vi "Proj3_Wireless_DTMF_Transmitter.vi"(6 "Gray Bit Encoding":bool, 7 "Dial Tone":bool, 8 "Quantization Level":u16(ring)=4 items=["2"=2, "4"=4, "8"=8, "16"=16], 9 "Phone # String":string) -> (0 "In Transmission":bool, 1 "bitLength":i32, 2 "quants":dbl[](array[numeric]), 3 "TXbitStream":i8[](array[numeric]), 4 "TX DTMF Signal":dbl[][](array[numeric]))   [LabVIEW 2011]
panel:
  out "Transmitted DTMF Signal":dbl[][](graph)
  in  "Tab Control":enum32{"DTMF", "Quantization"}(tab)
  in  "OK Button":bool
  in  "Snapshot Run":bool=TRUE
  # "Project 3: Wireless DTMF Transmitter"
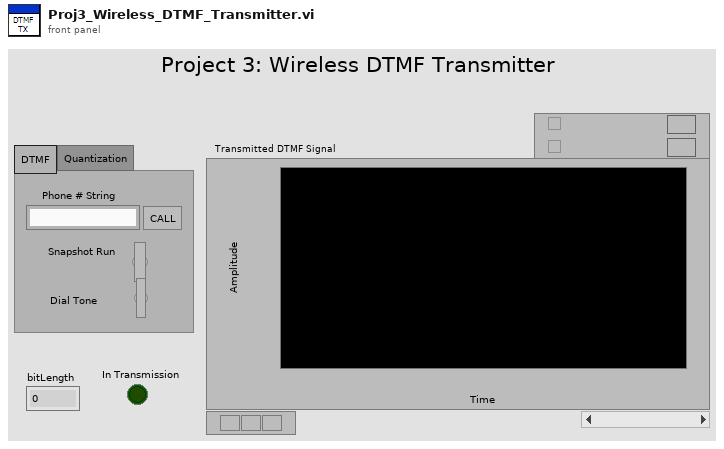
[diagram p1: front panel]
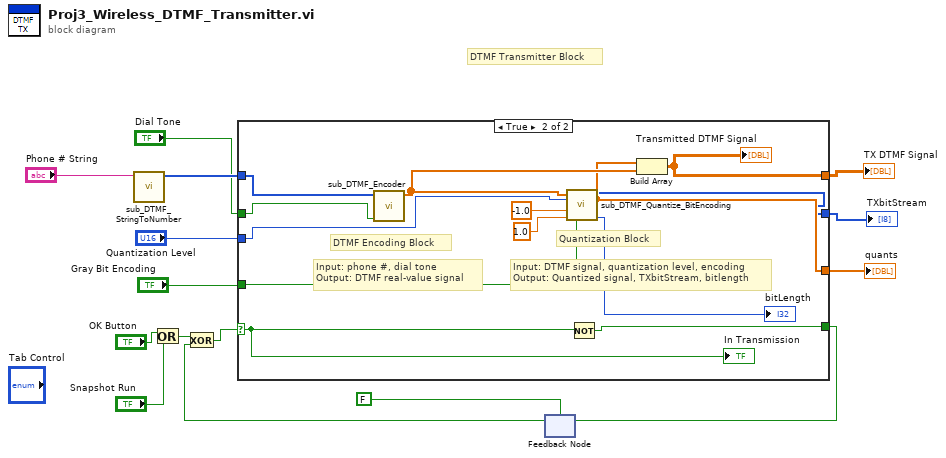
[diagram p0: block diagram]
diagram:
  # "DTMF Transmitter Block"
  n1 = call "sub_DTMF_StringToNumber.vi"("Phone # String"="Phone # String") -> ("Phone Number"=w12:u8[])  [unwired: 10 in]
  n2 = Or(x="OK Button", y="Snapshot Run") -> (x .or. y?=w8:bool)
  n3 = feedback #1(FALSE) -> (w14:bool)
  n4 = Exclusive Or(1:w14, 2:w8) -> (0:w3:bool)
  n5 = case shown="True" w3 {
    selector: w3 -> [_ w17]
    tunnel: w12 -> [_ w28]
    tunnel: "Quantization Level" -> [_ w27]
    tunnel: "Gray Bit Encoding" -> [_ w26]
    tunnel: [_ w22] -> w2
    tunnel: [_ w20] -> w7
    tunnel: [_ w19] -> w6
    tunnel: "Dial Tone" -> [_ w18]
    tunnel: [_ w16] -> w1
    frame False {
    }
    frame True {
      # "Input: DTMF signal, quantization level, encoding\nOutput: Quantized signal, TXbitStream, bitlength"
      # "Quantization Block"
      # "Input: phone #, dial tone\nOutput: DTMF real-value signal"
      # "DTMF Encoding Block"
      n6 = call "sub_DTMF_Encoder.vi"("Dial Tone"=w18, "digits"=w28) -> ("signal"=w23:dbl[])  [unwired: 9 in]
      n7 = call "sub_DTMF_Quantize_BitEncoding.vi"("signal"=w23, "L"=w27, "xmin"=-1.0, "xmax"=1.0, "GrayCode"=w26) -> ("TXbitStream"=w19:i32[], "quants"=w20:dbl[], "bitLength"=→"bitLength":i32)  [unwired: 6 in, 2 out]
      n8 = Not(x=w17) -> (.not. x?=w22:bool)
      n9 = Build Array(w20, w23) -> (w16:dbl[][])
      "Transmitted DTMF Signal" <- w16
      "In Transmission" <- w17
    }
  }
  "quants" <- w7
  "TXbitStream" <- w6
  "TX DTMF Signal" <- w1
  n10 = feedback-in #1(w2) -> ()
